vi "optagefrekvenssignal0.5.vi"() -> ()   [LabVIEW 2014]
uses:
  <vilib>/measure/maspectr.llb/FFT Power Spectrum and PSD for 1 Chan.vi
  <vilib>/measure/NI_MAPro.lvlib
panel:
  out "Array":dbl[](array[numeric])
  in  "Tid":dbl
  out "Maks frekvens":dbl
  out "FFT af lydsignal":dbl[](graph)
  out "Lydsignal":waveform(dbl)(graph)
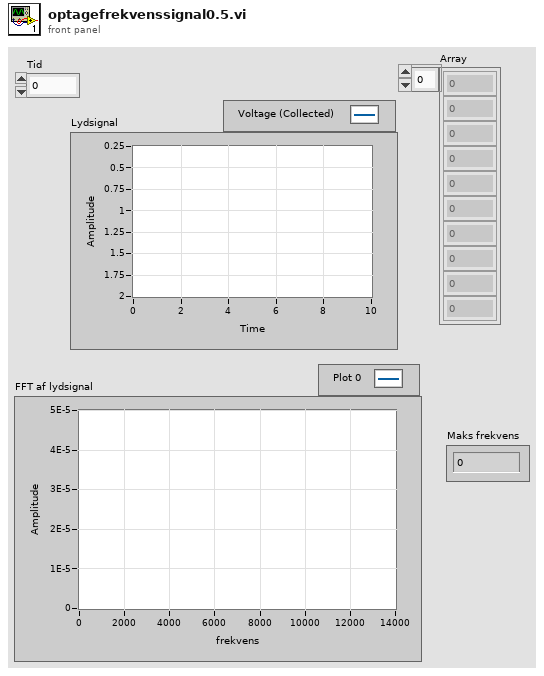
[diagram p1: front panel]
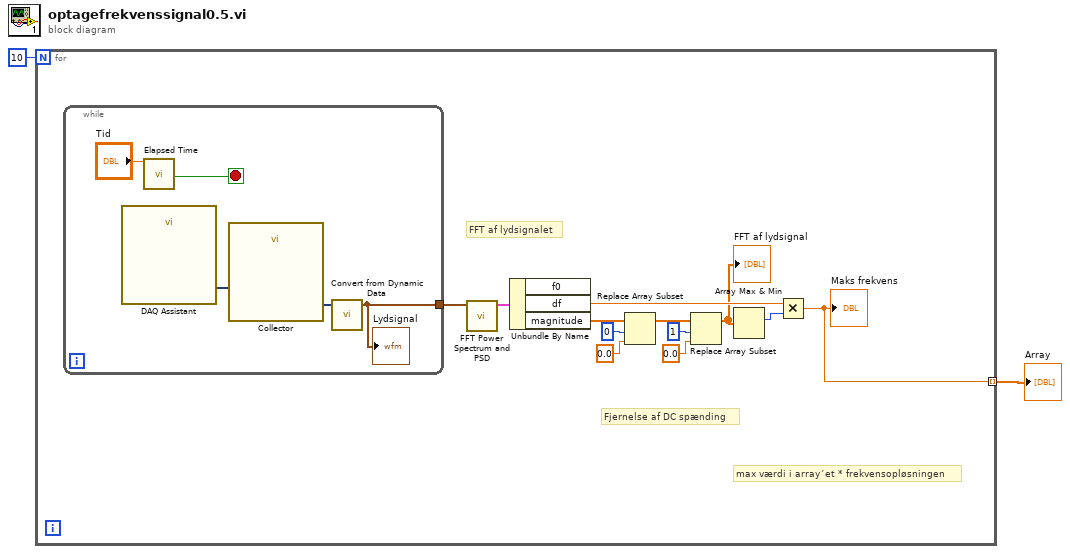
[diagram p0: block diagram]
diagram:
  n1 = for {
    N: 10 -> [_]
    tunnel: [w3] -> w1 mode=indexing
    # "max værdi i array´et * frekvensopløsningen"
    # "Fjernelse af DC spænding"
    # "FFT af lydsignalet"
    n2 = while {
      tunnel: [w19] -> w14
      stop <- w15 stop-if-true
      n3 = call "DAQ Assistant"() -> ("data"=w18:dynamicdata)  [unwired: 17 in, 2 out]
      n4 = call "Elapsed Time"("Time Target (s)"="Tid") -> ("Time has Elapsed"=w15:bool)  [unwired: 11 in, 7 out]
      n5 = call "Collector"("Signals"=w18) -> ("Collected Signals"=w17:dynamicdata)  [unwired: 9 in, 1 out]
      n6 = call "Convert from Dynamic Data"("Dynamic Data Type"=w17) -> ("Waveform"=w19:waveform(dbl))  [unwired: 3 in]
      "Lydsignal" <- w19
    }
    n7 = call-poly <vilib>:"FFT Power Spectrum and PSD.vi"("time signal"=w14) -> ("Power Spectrum / PSD"=w6:cluster{"f0":dbl, "df":dbl, "magnitude":dbl[]})  [unwired: 7 in, 3 out]
    n8 = Unbundle By Name(w6) -> ("df"=w7:dbl, "magnitude"=w5:dbl[])  [unwired: 1 out]
    n9 = Replace Array Subset(array=w5, new element=0.0 ("new element/subarray"), index=0) -> (w11:dbl[])
    n10 = Replace Array Subset(array=w11, new element=0.0 ("new element/subarray"), index=1) -> (w4:dbl[])
    "FFT af lydsignal" <- w4
    n11 = Array Max & Min(array=w4) -> (max index (indices)=w8:i32)  [unwired: 3 out]
    n12 = Multiply(x=w7, y=w8) -> (x*y=w3:dbl)
    "Maks frekvens" <- w3
  }
  "Array" <- w1
